vi "Analysis.Build List of Unique Items, Int32.vi"(10 "Item In":i32, 11 "List In":i32[](array[numeric])) -> (2 "Added":bool, 3 "List Out":i32[](array[numeric]), 5 "Index":i32)   [LabVIEW 2024]
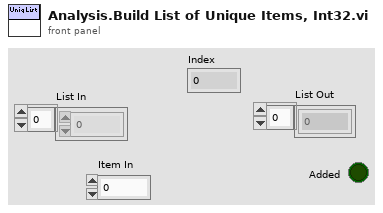
[diagram p1: front panel]
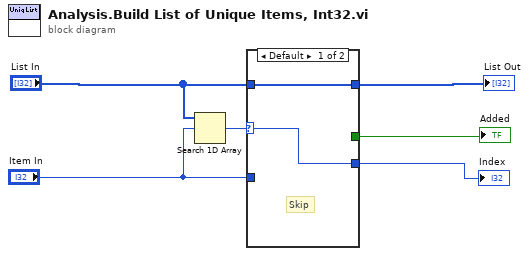
[diagram p0: block diagram]
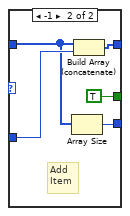
[diagram p2: hidden frame]
diagram:
  n1 = Search 1D Array(1D array="List In", element="Item In") -> (index of element=w3:i32)  [unwired: 1 in]
  n2 = case shown="Default" w3 {
    selector: w3 -> [w7 _]
    tunnel: "Item In" -> [_ w12]
    tunnel: "List In" -> [w8 w10]
    tunnel: [w8 w13] -> w5
    tunnel: [_ TRUE] -> w2
    tunnel: [w7 w9] -> w1
    frame Default {
      # "Skip"
    }
    frame -1 {
      # "Add\nItem"
      n3 = Array Size(array=w10) -> (size(s)=w9:i32)
      n4 = Build Array (concatenate)(w10, w12) -> (w13:i32[])
    }
  }
  "List Out" <- w5
  "Added" <- w2
  "Index" <- w1
